vi "Edit_Channel_Panel.vi"(0 "All Channel names":string[](array[string])=["30-10-03:New:Channel new5"], 9 "Result files to read":path[](array[path]), 11 "Selected Row":i32) -> (3 "New Values Out":string[](array[string])=["Test data5"], 4 "New Chs Out":string[](array[string])=["30-10-03:New:Channel new5"], 6 "Cancel Out":bool, 8 "Edit Raw Data Header Info Out":bool, 10 "Plotted rows only?":bool, 12 "Selected Row?":bool, 13 "Edit Raw data files?":bool, 14 "Raw data files in Orig Positions?":bool, 15 "Mode":T1)   [LabVIEW 2016]
uses:
  Plotter_Mode.ctl
panel:
  in  "Select channel names":bool
  in  "Cancel":bool
  in  "Edit Raw data files":i32(listbox)=1
  in  "Columns to Output":i32[](listbox)
  in  "Edit Type":i32(listbox)
  in  "OK Button":bool
  in  "Add values to:":i32(listbox)=1
  in  "New Values In":string[](array[string])=["Value"]
  in  "New Chs In":string[](array[string])=["Channel Name"]
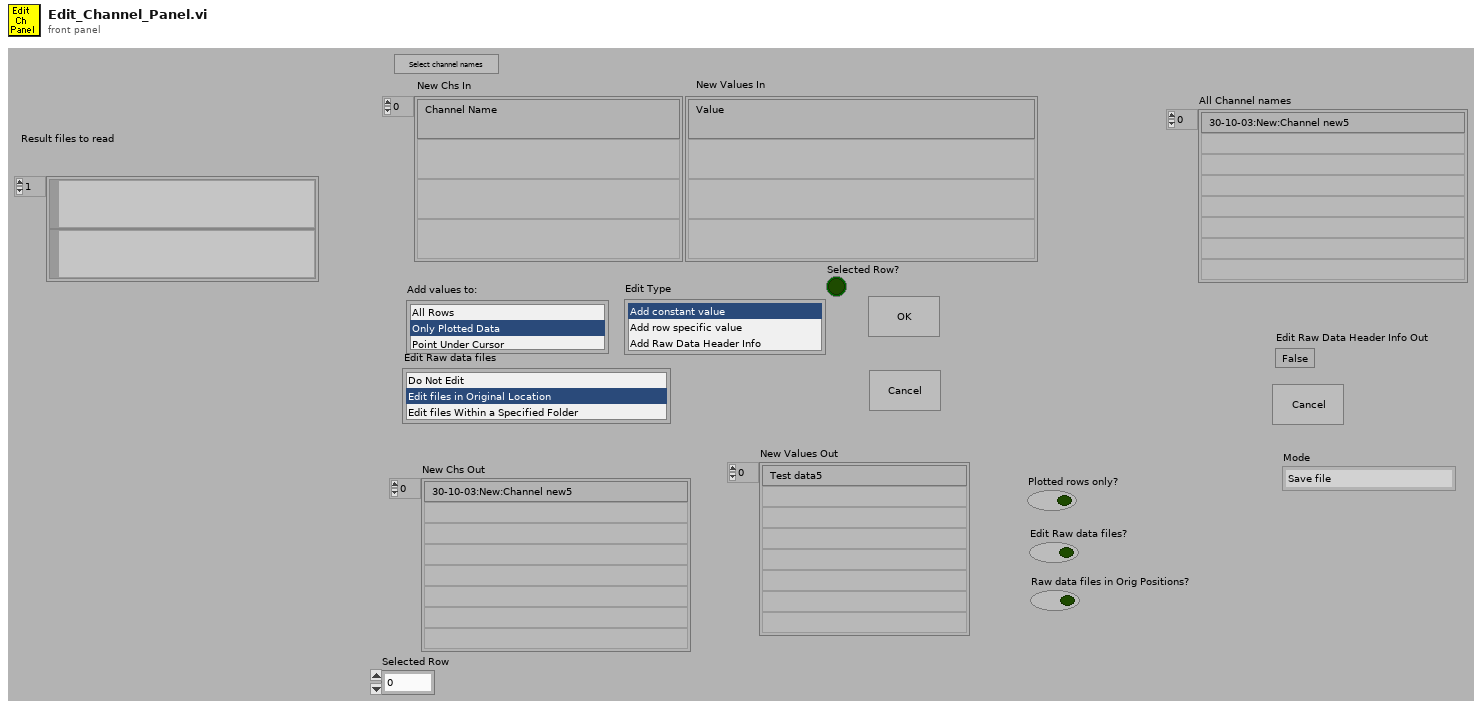
[diagram p1: front panel]
types:
  T1 = typedef "Plotter_Mode.ctl" = enum16{"Save file", "Delete unwanted rows", "Edit Values with constants", "Edit values per row", "Edit Raw Data file header", "Post Process Plotted Rows", "Plot EnFlo Tunnel Display", "Add Inlet Temperature Offset"}
  T2 = enum16{"Read Channels From File", "Read Channels from Server"}
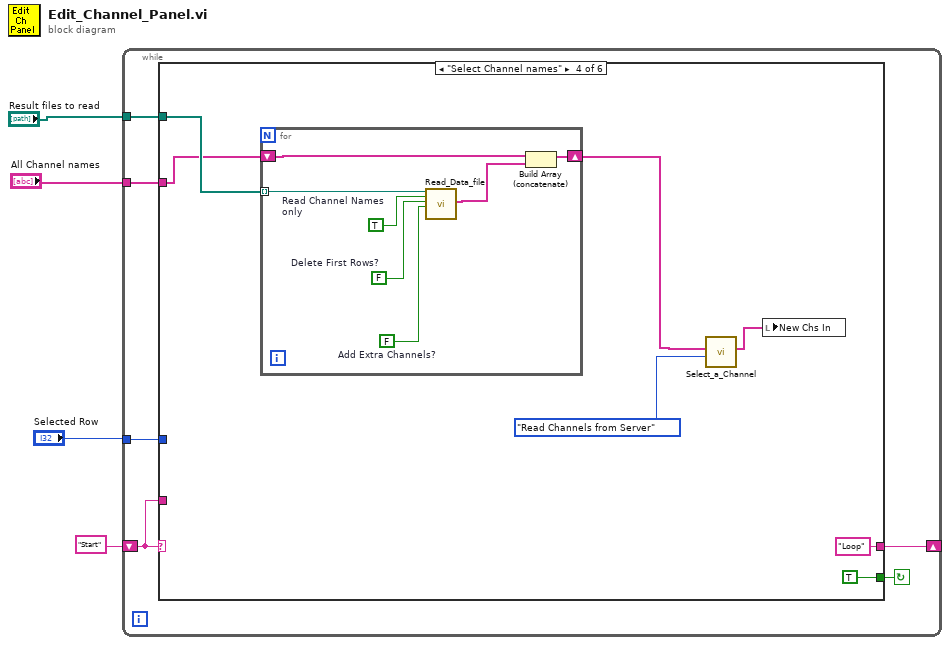
[diagram p0: block diagram]
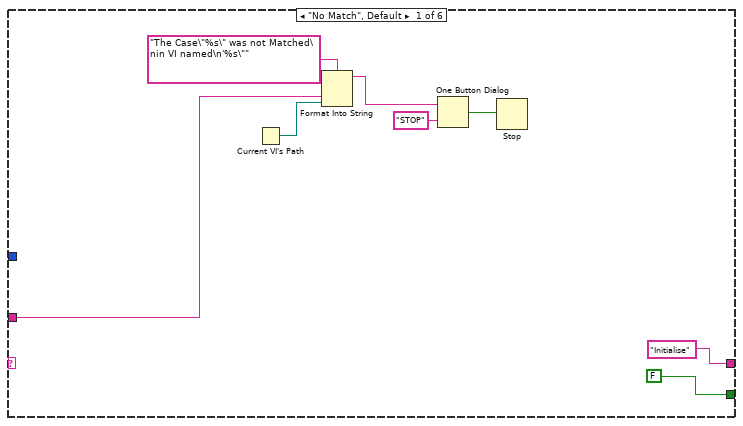
[diagram p2: hidden frame]
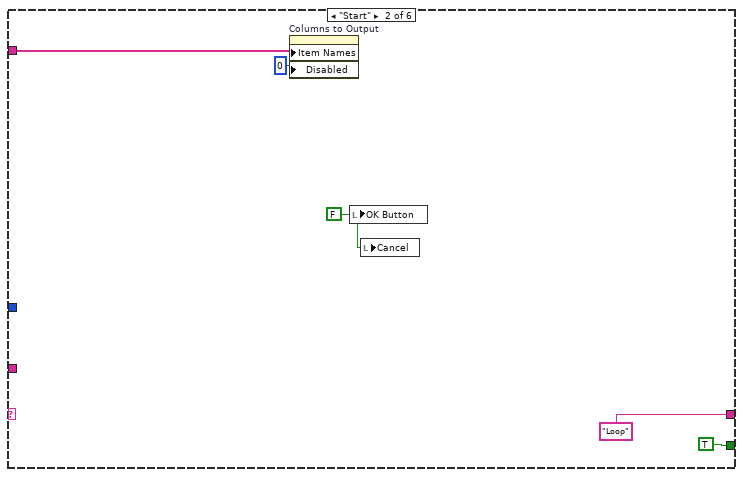
[diagram p3: hidden frame]
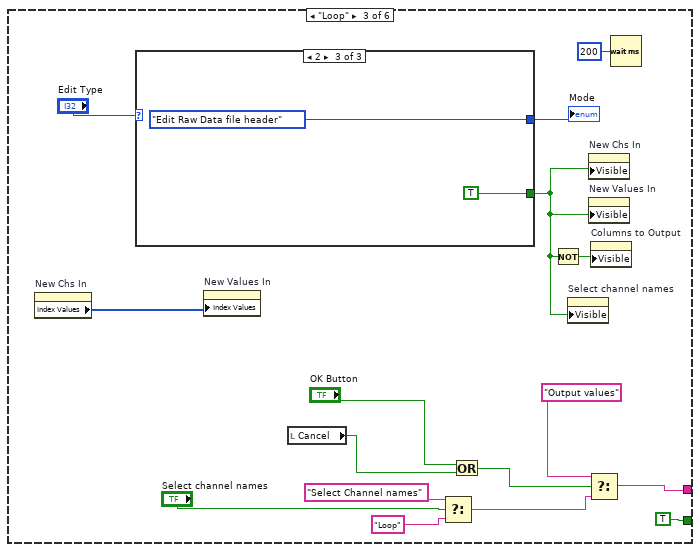
[diagram p4: hidden frame]
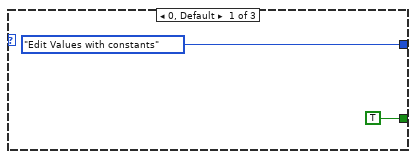
[diagram p5: hidden frame]
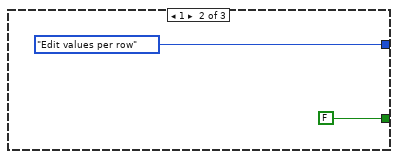
[diagram p6: hidden frame]
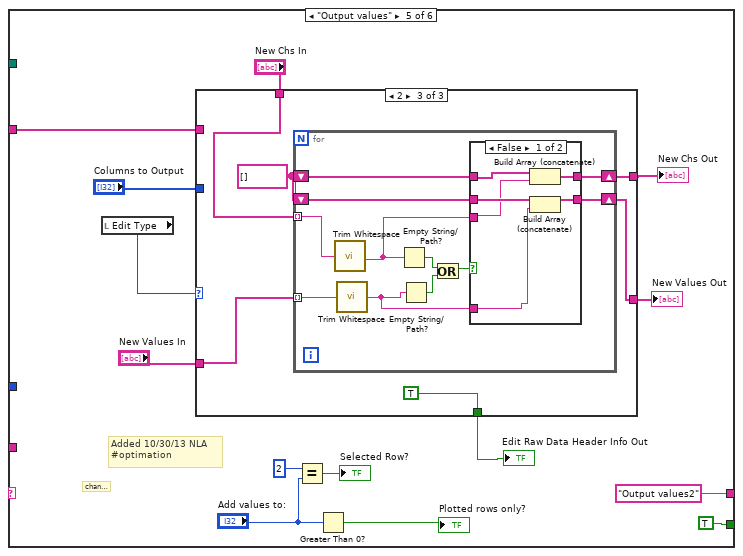
[diagram p7: hidden frame]
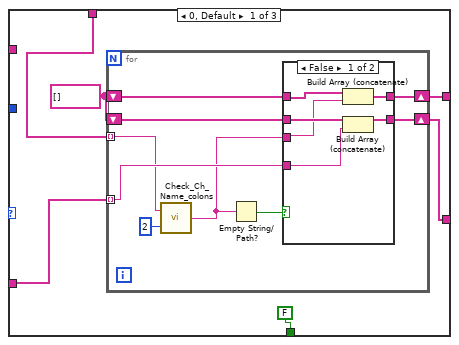
[diagram p8: hidden frame]
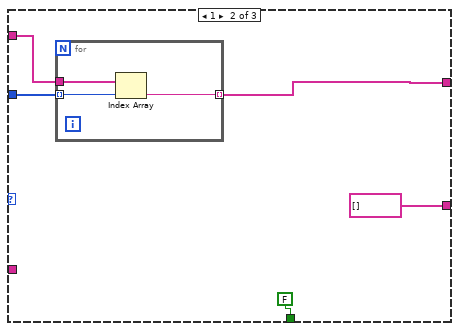
[diagram p10: hidden frame]
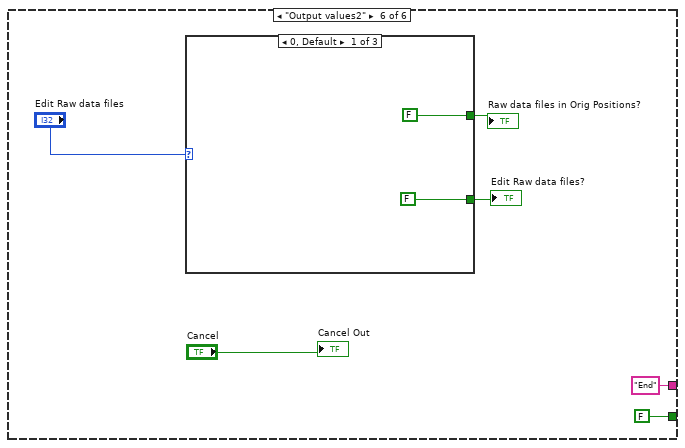
[diagram p12: hidden frame]
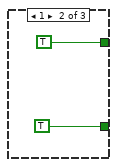
[diagram p13: hidden frame]
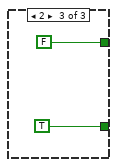
[diagram p14: hidden frame]
diagram:
  n1 = while {
    shift-left: "Start" -> [w8]
    shift-right: [w9] -> _
    tunnel: "All Channel names" -> [w7]
    tunnel: "Result files to read" -> [w6]
    tunnel: "Selected Row" -> [w5]
    stop <- w10 continue-if-true
    n2 = case shown="\"Select Channel names\"" w8 {
      tunnel: [FALSE TRUE TRUE TRUE TRUE FALSE] -> w10
      tunnel: ["Initialise" "Loop" w37 "Loop" "Output values2" "End"] -> w9
      tunnel: w8 -> [w13 _ _ _ _ _]
      tunnel: w7 -> [_ w21 _ w50 w64 _]
      tunnel: w6 -> [_ _ _ w51 _ _]
      tunnel: w5 -> [_ _ _ _ _ _]
      frame "No Match", Default {
        n3 = Current VI's Path() -> (path=w12:path)
        n4 = Format Into String(format string="The Case\"%s\" was not Matched\nin VI named\n'%s\"" ("Format String"), w13, w12) -> (resulting string=w16:string)  [unwired: 2 in, 1 out]
        n5 = One Button Dialog(message=w16, button name ("OK")="STOP") -> (true=w14:bool)
        n6 = Stop(stop? (T)=w14) -> ()
      }
      frame "Start" {
        w19 = FALSE ("OK Button")
        n7 = property on="Columns to Output" class="LstBox (strict)"("Item Names"=w21, "Disabled"=u8 0) -> ()  [unwired: 2 in, 2 out]
        n8 = local write "OK Button"(w19) -> ()
        n9 = local write "Cancel"(w19) -> ()
      }
      frame "Loop" {
        n10 = property on="New Chs In" class="Arr (strict)"() -> ("Index Values"=w27:u32[])  [unwired: 2 in, 2 out]
        n11 = case shown="2" "Edit Type" {
          tunnel: [Plotter_Mode."Edit Values with constants" ("Mode") Plotter_Mode."Edit values per row" ("Mode") Plotter_Mode."Edit Raw Data file header" ("Mode")] -> w35
          tunnel: [TRUE FALSE TRUE] -> w24
          frame 0, Default {
          }
          frame 1 {
          }
          frame 2 {
          }
        }
        "Mode" <- w35
        n12 = property on="New Values In" class="Arr (strict)"("Index Values"=w27) -> ()  [unwired: 2 in, 2 out]
        n13 = local read "Cancel"() -> (w33:bool)
        n14 = Select(t="Select Channel names", s="Select channel names", f="Loop") -> (s? t:f=w26:string)
        n15 = Or(x="OK Button", y=w33) -> (x .or. y?=w31:bool)
        n16 = Not(x=w24) -> (.not. x?=w34:bool)
        n17 = property on="Select channel names" class="Bool"("Visible"=w24) -> ()  [unwired: 2 in, 2 out]
        n18 = property on="New Chs In" class="Arr (strict)"("Visible"=w24) -> ()  [unwired: 2 in, 2 out]
        n19 = property on="New Values In" class="Arr (strict)"("Visible"=w24) -> ()  [unwired: 2 in, 2 out]
        n20 = Select(t="Output values", s=w31, f=w26) -> (s? t:f=w37:string)
        n21 = property on="Columns to Output" class="LstBox (strict)"("Visible"=w34) -> ()  [unwired: 2 in, 2 out]
        n22 = Wait (ms)(milliseconds to wait=u32 200) -> ()  [unwired: 1 out]
      }
      frame "Select Channel names" {
        n23 = for {
          shift-right: [w57] -> w49
          shift-left: w50 -> [w55]
          tunnel: w51 -> [w59] mode=indexing
          w53 = FALSE  # Delete First Rows?
          w54 = FALSE  # Add Extra Channels?
          w58 = TRUE  # Read Channel Names only
          n24 = call "Read_Data_file.vi"("Results file"=w59, "Read Channel Names only"=w58, "Delete First Rows?"=w53, "Add Extra Channels?"=w54) -> ("Ch names Out"=w56:string[])  [unwired: 3 in, 12 out]
          n25 = Build Array (concatenate)(w55, w56) -> (w57:string[])
        }
        n26 = call "Select_a_Channel.vi"("Mode"=T2."Read Channels from Server", "Extra channel names"=w49) -> ("Selected Channel Names"=w48:string[])  [unwired: 1 in, 5 out]
        n27 = local write "New Chs In"(w48) -> ()
      }
      frame "Output values" {
        # "Added 10/30/13 NLA\n#optimation"
        # "channel"
        n28 = local read "Edit Type"() -> (w70:i32)
        n29 = case shown="2" w70 {
          tunnel: "New Values In" -> [w77 _ w108]
          tunnel: [w76 string[] [] w107] -> w68
          tunnel: "New Chs In" -> [w78 _ w109]
          tunnel: [w75 w99 w106] -> w66
          tunnel: "Columns to Output" -> [_ w101 _]
          tunnel: w64 -> [_ w100 _]
          tunnel: [FALSE FALSE TRUE] -> w63
          frame 0, Default {
            w79 = string[] []
            n30 = for {
              tunnel: w77 -> [w84] mode=indexing
              shift-right: [w85] -> w75
              shift-left: w79 -> [w88]
              shift-right: [w87] -> w76
              shift-left: w79 -> [w86]
              tunnel: w78 -> [w83] mode=indexing
              n31 = call "Check_Ch_Name_colons.vi"("No of Colons"=2, "Ch Name in"=w83) -> ("Ch Name out"=w82:string)
              n32 = Empty String/Path?(string/path=w82) -> (empty?=w81:bool)
              n33 = case shown="False" w81 {
                tunnel: [w91 w96] -> w85
                tunnel: w88 -> [w94 w96]
                tunnel: [w92 w95] -> w87
                tunnel: w86 -> [w93 w95]
                tunnel: w84 -> [w89 _]
                tunnel: w82 -> [w90 _]
                frame False {
                  n34 = Build Array (concatenate)(w94, w90) -> (w91:string[])
                  n35 = Build Array (concatenate)(w93, w89) -> (w92:string[])
                }
                frame True {
                }
              }
            }
          }
          frame 1 {
            n36 = for {
              tunnel: w101 -> [w104] mode=indexing
              tunnel: w100 -> [w103]
              tunnel: [w102] -> w99 mode=indexing
              n37 = Index Array(array=w103, index=w104) -> (element=w102:string)
            }
          }
          frame 2 {
            w110 = string[] []
            n38 = for {
              tunnel: w108 -> [w116] mode=indexing
              shift-right: [w118] -> w106
              shift-left: w110 -> [w121]
              shift-right: [w120] -> w107
              shift-left: w110 -> [w119]
              tunnel: w109 -> [w117] mode=indexing
              n39 = call <vilib>:"Trim Whitespace.vi"("string"=w117) -> ("trimmed string"=w112:string)  [unwired: 1 in]
              n40 = call <vilib>:"Trim Whitespace.vi"("string"=w116) -> ("trimmed string"=w111:string)  [unwired: 1 in]
              n41 = Empty String/Path?(string/path=w112) -> (empty?=w114:bool)
              n42 = Empty String/Path?(string/path=w111) -> (empty?=w115:bool)
              n43 = Or(x=w114, y=w115) -> (x .or. y?=w113:bool)
              n44 = case shown="False" w113 {
                tunnel: [w124 w129] -> w118
                tunnel: w121 -> [w127 w129]
                tunnel: [w125 w128] -> w120
                tunnel: w119 -> [w126 w128]
                tunnel: w112 -> [w123 _]
                tunnel: w111 -> [w122 _]
                frame False {
                  n45 = Build Array (concatenate)(w127, w123) -> (w124:string[])
                  n46 = Build Array (concatenate)(w126, w122) -> (w125:string[])
                }
                frame True {
                }
              }
            }
          }
        }
        "New Values Out" <- w68
        "New Chs Out" <- w66
        "Edit Raw Data Header Info Out" <- w63
        n47 = Equal?(x=2, y="Add values to:") -> (x = y?=→"Selected Row?":bool)
        n48 = Greater Than 0?(x="Add values to:") -> (x > 0?=→"Plotted rows only?":bool)
      }
      frame "Output values2" {
        n49 = case shown="0, Default" "Edit Raw data files" {
          tunnel: [FALSE TRUE TRUE] -> w132
          tunnel: [FALSE TRUE FALSE] -> w131
          frame 0, Default {
          }
          frame 1 {
          }
          frame 2 {
          }
        }
        "Edit Raw data files?" <- w132
        "Raw data files in Orig Positions?" <- w131
        "Cancel Out" <- "Cancel"
      }
    }
  }
